vi "getWavelength_v80.vi"() -> ()   [LabVIEW 2012]
uses:
  x32/CLDevIFace.dll
panel:
  out "error out":errorcluster
  out "output param":i32
  in  "stop":bool
  in  "OK Button":bool
  out "Wavelength":dbl format="%.9f"
  in  "CommPort":dbl caption="Comm Port #"
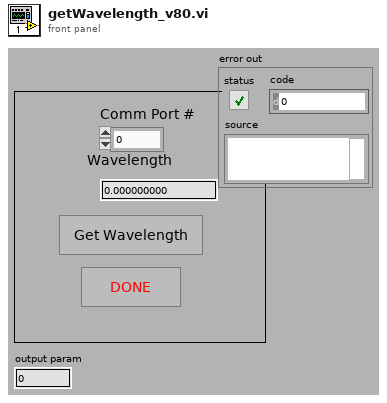
[diagram p1: front panel]
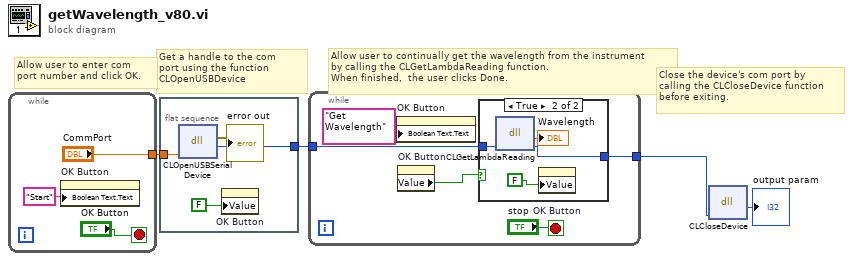
[diagram p0: block diagram]
diagram:
  # "Close the device's com port by\ncalling the CLCloseDevice function\nbefore exiting."
  # "Allow user to continually get the wavelength from the instrument\nby calling the CLGetLambdaReading function.  \nWhen finished,  the user clicks Done."
  # "Get a handle to the com\nport using the function CLOpenUSBDevice"
  # "Allow user to enter com \nport number and click OK."
  n1 = while {
    tunnel: ["CommPort"] -> w4
    stop <- "OK Button" stop-if-true
    n2 = property on="OK Button" class="Bool (strict)"("Boolean Text.Text"="Start") -> ()  [unwired: 2 in, 2 out]
  }
  n3 = flat-sequence {
    tunnel: w4 -> [w11]
    tunnel: [w10] -> w3
    frame #0 {
      n4 = dll-call lib="C:/Users/Lab/Desktop/Bristol wavemeter 621/00424-2-00 621 customer CD/Programming Interface/x32/CLDevIface.dll" fn="CLOpenUSBSerialDevice"("commPort"=w11) -> (error out=→"error out":errorcluster, "return type"=w10:i32)  [unwired: 4 in, 1 out]
      n5 = property on="OK Button" class="Bool (strict)"("Value"=FALSE) -> ()  [unwired: 2 in, 2 out]
    }
  }
  n6 = while {
    tunnel: w3 -> [w16]
    tunnel: [w12] -> w2
    stop <- "stop" stop-if-true
    n7 = property on="OK Button" class="Bool (strict)"("Boolean Text.Text"="Get Wavelength") -> ()  [unwired: 2 in, 2 out]
    n8 = property on="OK Button" class="Bool (strict)"() -> ("Value"=w13:bool)  [unwired: 2 in, 2 out]
    n9 = case shown="True" w13 {
      tunnel: w16 -> [w17 w21]
      tunnel: [w17 w18] -> w12
      frame False {
      }
      frame True {
        n10 = dll-call lib="C:/Users/Lab/Desktop/Bristol wavemeter 621/00424-2-00 621 customer CD/Programming Interface/x32/CLDevIface.dll" fn="CLGetLambdaReading"("devHandle"=w21) -> ("return type"=→"Wavelength":dbl, "devHandle"=w18:i32)  [unwired: 3 in, 2 out]
        n11 = property on="OK Button" class="Bool (strict)"("Value"=FALSE) -> ()  [unwired: 2 in, 2 out]
      }
    }
  }
  n12 = dll-call lib="C:/Users/Lab/Desktop/Bristol wavemeter 621/00424-2-00 621 customer CD/Programming Interface/x32/CLDevIface.dll" fn="CLCloseDevice"("commPort"=w2) -> ("return type"=→"output param":i32)  [unwired: 4 in, 2 out]
